vi "Fix_Metadata.vi"(11 "Array in":string[](array[string])) -> (3 "Array out":string[](array[string]))   [LabVIEW 2016]
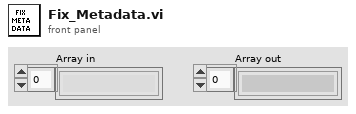
[diagram p1: front panel]
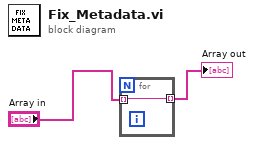
[diagram p0: block diagram]
diagram:
  n1 = for {
    tunnel: "Array in" -> [w3] mode=indexing
    tunnel: [w3] -> w2 mode=indexing
  }
  "Array out" <- w2
